vi "2D FFT Example.vi"() -> ()   [LabVIEW 2012]
uses:
  Non-User VIs/Error Checking/View Error Log Mode Functional Global.vi
  OpenCLV x64.lvlib
panel:
  out "Labview Real":dbl[][](array[numeric])
  out "Labview Imag":dbl[][](array[numeric])
  out "OpenCLV Imag":dbl[][](array[numeric])
  out "OpenCLV Real":dbl[][](array[numeric])
  out "OpenCLV Time":u32
  out "Labview Time":u32
  in  "FFT Dimension":enum16{"1D FFT", "2D FFT"}(ring)=enum."2D FFT"
  in  "Dimension":cluster{"Depth":u64, "Height":u64, "Width":u64}={"Depth"=1, "Height"=1000, "Width"=1024} {"Width" min=1; "Height" min=1; "Depth" min=1}
  # "Outputs"
  # "Inputs - Change before running"
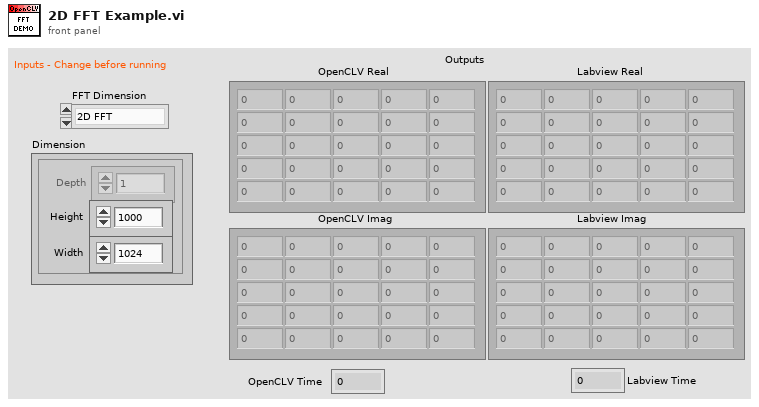
[diagram p1: front panel]
types:
  T1 = enum16{"Allocate", "Compute FFT and IFFT", "Compute Labivew FFT and IFFT", "Clean up"}
  T2 = typedef "OpenCLV x64.lvlib/Device ID.ctl" = u64
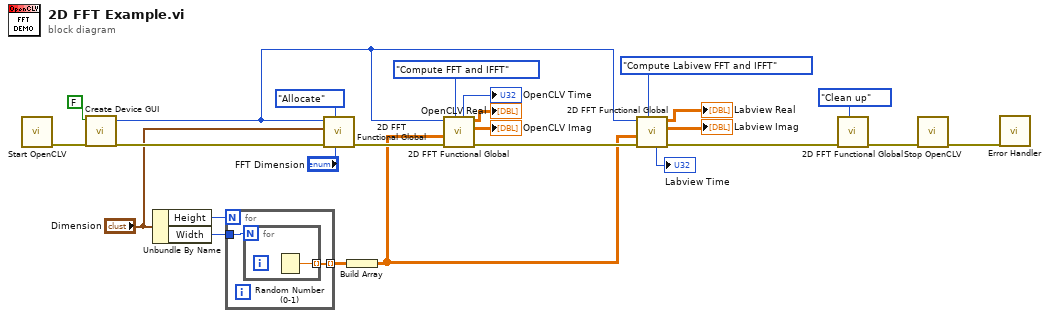
[diagram p0: block diagram]
diagram:
  n1 = call "Start OpenCLV.vi"() -> ("Error Out"=w22:errorcluster)  [unwired: 11 in]
  n2 = call "Create Device GUI.vi"("Error In"=w22, "Skip Configuration"=FALSE) -> ("error constant"=w21:errorcluster, "Device Reference"=w13:T2)  [unwired: 8 in]
  n3 = Unbundle By Name("Dimension") -> ("Height"=w24:u64, "Width"=w23:u64)
  n4 = for {
    N: w24 -> [_]
    tunnel: w23 -> [w27]
    tunnel: [w26] -> w15 mode=indexing
    n5 = for {
      N: w27 -> [_]
      tunnel: [w28] -> w26 mode=indexing
      n6 = Random Number (0-1)() -> (number: 0 to 1=w28:dbl)
    }
  }
  n7 = call "2D FFT Functional Global.vi"("FFT Dimension"="FFT Dimension", "FFT States"=T1."Allocate", "Error In"=w21, "Dimension FFT"="Dimension", "Device"=w13) -> ("Error Out"=w16:errorcluster)  [unwired: 2 in, 4 out]
  n8 = Build Array(w15) -> (w12:dbl[][][])
  n9 = call "2D FFT Functional Global.vi"("FFT States"=T1."Compute FFT and IFFT", "Error In"=w16, "Real In"=w12, "Device"=w13) -> ("Error Out"=w14:errorcluster, "Imag Data"=→"OpenCLV Imag":dbl[][], "Real Data"=→"OpenCLV Real":dbl[][], "OpenCLV Time"=→"OpenCLV Time":u32)  [unwired: 3 in, 1 out]
  n10 = call "2D FFT Functional Global.vi"("FFT States"=T1."Compute Labivew FFT and IFFT", "Error In"=w14, "Real In"=w12, "Device"=w13) -> ("Error Out"=w8:errorcluster, "Imag Data"=→"Labview Imag":dbl[][], "Real Data"=→"Labview Real":dbl[][], "Labview Time"=→"Labview Time":u32)  [unwired: 3 in, 1 out]
  n11 = call "2D FFT Functional Global.vi"("FFT States"=T1."Clean up", "Error In"=w8) -> ("Error Out"=w6:errorcluster)  [unwired: 5 in, 4 out]
  n12 = call "Stop OpenCLV.vi"("Error In"=w6) -> ("Error Out"=w5:errorcluster)  [unwired: 10 in]
  n13 = call-poly "Error Handler.vi"("Error In"=w5) -> ()  [unwired: 10 in, 1 out]
